vi "Interpolate 1D Complex Double Array.vi"(1 "xi":dbl[](array[numeric]), 2 "X":dbl[](array[numeric]), 3 "Y":cdb[](array[numeric])) -> (0 "yi":cdb[](array[numeric]))   [LabVIEW 2023, in "NI_HFNetworkAnalysis.lvlib"]
doc: "Performs one-dimensional interpolation of complex double-precision floating-point values, using a spline method, based on the lookup table defined by X and Y.\n\n<b>Remarks:</b>\nThe X array of the lookup table is assumed monotonic."
uses:
  NI_HFNetworkAnalysis.lvlib
  <vilib>/gmath/NI_Gmath.lvlib
  <vilib>/Analysis/NI_AALPro.lvlib
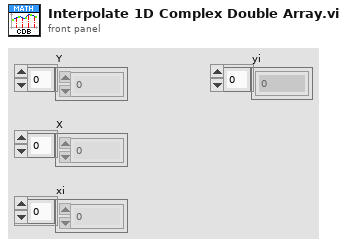
[diagram p1: front panel]
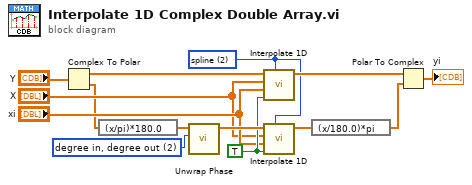
[diagram p0: block diagram]
diagram:
  w8 = 2 items=["nearest", "linear", "spline", "cubic Hermite", "Lagrange"] ("method")
  w13 = TRUE ("X is monotonic")
  w3 = 2 items=["radian in, radian out", "radian in, degree out", "degree in, degree out", "degree in, radian out"] ("phase unit")
  n1 = Complex To Polar(r * e^(i*theta)="Y") -> (r=w5:dbl[], theta=w4:dbl[])
  n2 = expression code="(x/pi)*180.0" ("radians to degrees")(w4) -> (w2:dbl[])
  n3 = call <vilib>:"Unwrap Phase.vi"("phase unit"=w3, "Phase"=w2) -> ("Unwrapped Phase"=w14:dbl[])  [unwired: 8 in, 1 out]
  n4 = call <vilib>:"Interpolate 1D.vi"("method"=w8, "X is monotonic"=w13, "xi"="xi", "X"="X", "Y"=w5) -> ("yi"=w11:dbl[])  [unwired: 4 in, 2 out]
  n5 = call <vilib>:"Interpolate 1D.vi"("method"=w8, "X is monotonic"=w13, "xi"="xi", "X"="X", "Y"=w14) -> ("yi"=w9:dbl[])  [unwired: 4 in, 2 out]
  n6 = expression code="(x/180.0)*pi" ("degrees to radians")(w9) -> (w10:dbl[])
  n7 = Polar To Complex(1:w10, 2:w11) -> (0:→"yi":cdb[])
